vi "AppendTableToReport_Mutation.vi"(0 "Diagram":refnum<vi>, 5 "ObjRef":refnum<vi>, 6 "Kind":string="SubVI", 7 "Information":string="<Not A Path>") -> (3 "Replace?":bool)   [LabVIEW 2020]
uses:
  <vilib>/Utility/Data Type/NI_Data Type.lvlib
  <vilib>/Utility/Data Type/Type Definitions/Data Type.ctl
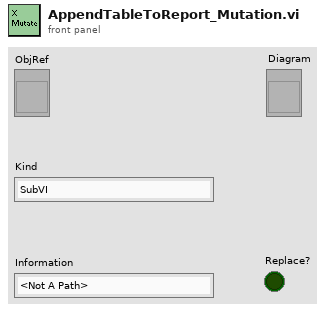
[diagram p1: front panel]
types:
  T1 = typedef "NI_Data Type.lvlib/Data Type.ctl" = enum8{"Invalid Type", "Void", "I8", "I16", "I32", "I64", "U8", "U16", "U32", "U64", "Single Float", "Double Float", "Extended Float", "Single Complex", "Double Complex", "Extended Complex", "Enum U8", "Enum U16", "Enum U32", "Enum U64", "Single Float With Unit", "Double Float With Unit", "Extended Float With Unit", "Single Complex with Unit", "Double Complex with Unit", "Extended Complex with Unit", "Boolean", "String", "Path", "Picture", "Tag", "Array", "Cluster", "Variant", "LV Variant", "Waveform", "Timestamp", "Digital Waveform", "Digital Data", "ExpressData", "Refnum", "External Data", "VI", "Poly VI", "LabVIEW Class Instance", "Fixed Point", "Set Collection", "Map Collection"}
  T2 = typedef "LVPositionTypeDef.ctl" = cluster{"Left":i32, "Top":i32}
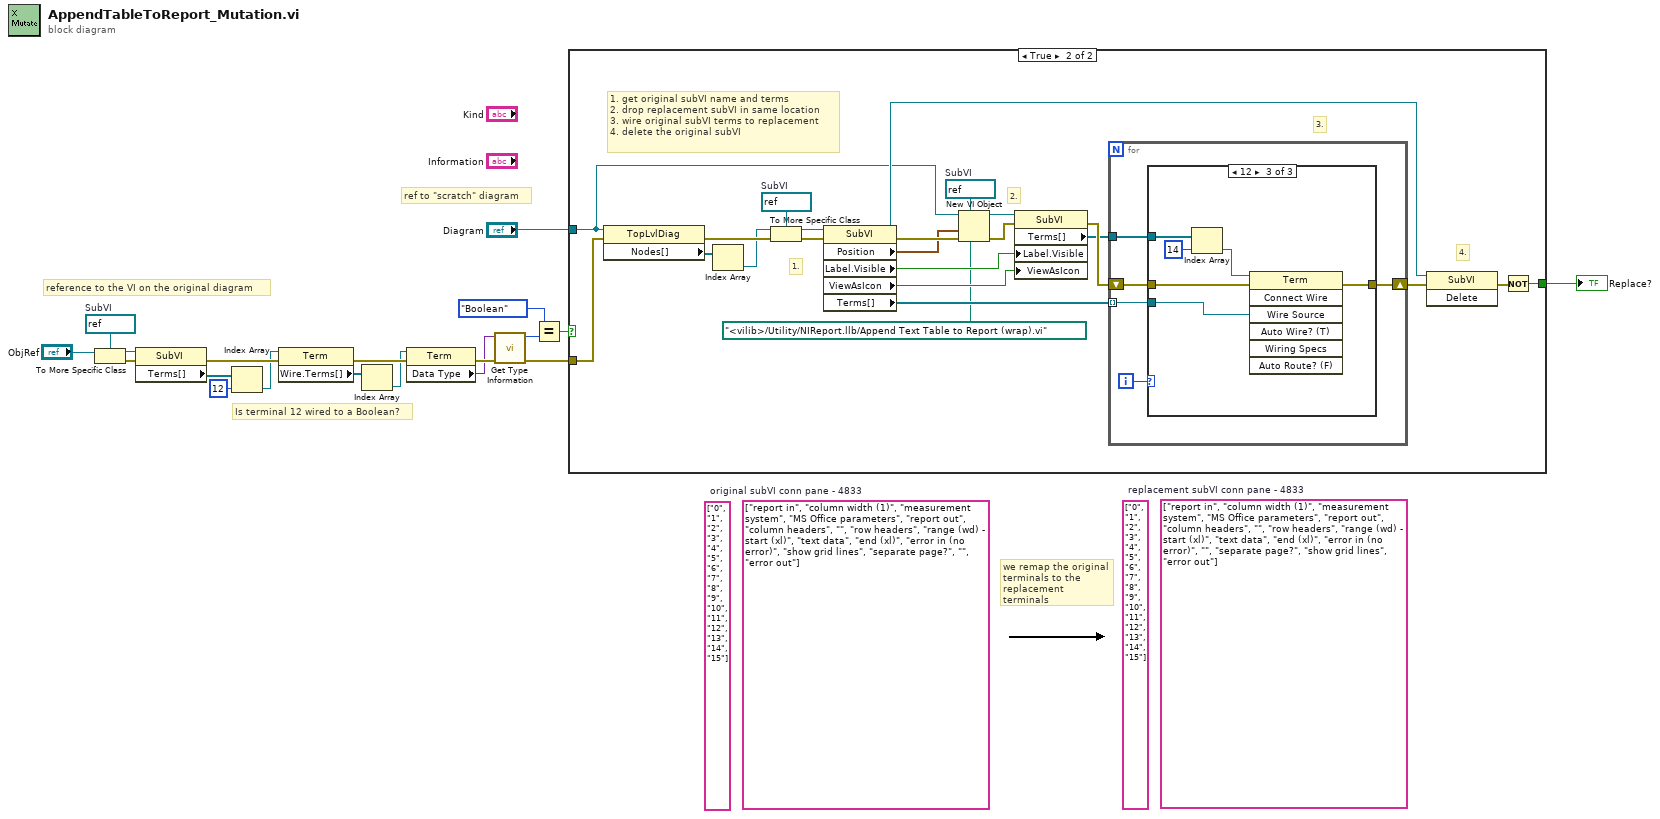
[diagram p0: block diagram]
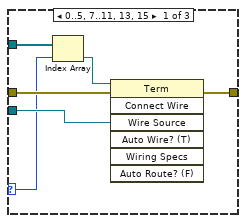
[diagram p3: hidden frame]
diagram:
  w12 = refnum<vi> refnum  # SubVI
  (unwired) string[] ["0", "1", "2", "3", "4", "5", "6", "7", "8", "9", "10", "11", "12", "13", "14", "15"]
  (unwired) string[] ["report in", "column width (1)", "measurement system", "MS Office parameters", "report out", "column headers", "", "row headers", "range (wd) - start (xl)", "text data", "end (xl)", "error in (no error)", "show grid lines", "separate page?", "", "error out"]  # original subVI conn pane - 4833
  (unwired) string[] ["0", "1", "2", "3", "4", "5", "6", "7", "8", "9", "10", "11", "12", "13", "14", "15"]
  (unwired) string[] ["report in", "column width (1)", "measurement system", "MS Office parameters", "report out", "column headers", "", "row headers", "range (wd) - start (xl)", "text data", "end (xl)", "error in (no error)", "", "separate page?", "show grid lines", "error out"]  # replacement subVI conn pane - 4833
  # "Is terminal 12 wired to a Boolean?"
  # "reference to the VI on the original diagram"
  # "we remap the original terminals to the replacement terminals"
  # "ref to \"scratch\" diagram"
  n1 = To More Specific Class(target class=w12, reference="ObjRef") -> (specific class reference=w10:refnum<vi>, error out=w19:errorcluster)  [unwired: 1 in]
  n2 = property class="SubVI"(reference=w10, error in=w19) -> (error out=w18:errorcluster, "Terms[]"=w9:refnum<vi>[])  [unwired: 1 out]
  n3 = Index Array(array=w9, index=12) -> (element=w7:refnum<vi>)
  n4 = property class="Term"(reference=w7, error in=w18) -> (error out=w17:errorcluster, "Wire.Terms[]"=w6:refnum<vi>[])  [unwired: 1 out]
  n5 = Index Array(array=w6) -> (element=w5:refnum<vi>)  [unwired: 1 in]
  n6 = property class="Term"(reference=w5, error in=w17) -> (error out=w16:errorcluster, "Data Type"=w4:variant)  [unwired: 1 out]
  n7 = call <vilib>:"Get Type Information.vi"("error in (no error)"=w16, "variant"=w4) -> ("error out"=w15:errorcluster, "type"=w3:T1)  [unwired: 5 in, 3 out]
  n8 = Equal?(x=Data_Type."Boolean", y=w3) -> (x = y?=w2:bool)
  n9 = case shown="True" w2 {
    tunnel: "Diagram" -> [_ w25]
    tunnel: [_ w24] -> w13
    tunnel: w15 -> [_ w35]
    frame False {
      # "If terminal 7 is not wired to a Boolean we do not need to rewire, because all the other terminals map the same."
    }
    frame True {
      w23 = refnum<vi> refnum  # SubVI
      w34 = refnum<vi> refnum  # SubVI
      # "4."
      # "3."
      # "2."
      # "1."
      # "1. get original subVI name and terms\n2. drop replacement subVI in same location\n3. wire original subVI terms to replacement\n4. delete the original subVI"
      n10 = property class="TopLvlDiag"(reference=w25, error in=w35) -> (error out=w42:errorcluster, "Nodes[]"=w33:refnum<vi>[])  [unwired: 1 out]
      n11 = Index Array(array=w33) -> (element=w32:refnum<vi>)  [unwired: 1 in]
      n12 = To More Specific Class(target class=w34, reference=w32, error in=w42) -> (specific class reference=w26:refnum<vi>, error out=w40:errorcluster)
      n13 = property class="SubVI"(reference=w26, error in=w40) -> (reference out=w30:refnum<vi>, error out=w41:errorcluster, "Position"=w29:T2, "Label.Visible"=w27:bool, "ViewAsIcon"=w28:bool, "Terms[]"=w31:refnum<vi>[])
      n14 = New VI Object(vi object class=w23, owner refnum=w25, position/next to=w29, 6:path "<vilib>/Utility/NIReport.llb/Append Text Table to Report (wrap).vi", 8:w41) -> (object refnum=w20:refnum<vi>, 0:w38:errorcluster)  [unwired: 3 in]
      n15 = property class="SubVI"(reference=w20, error in=w38, "Label.Visible"=w27, "ViewAsIcon"=w28) -> (error out=w37:errorcluster, "Terms[]"=w21:refnum<vi>[])  [unwired: 1 out]
      n16 = for {
        tunnel: w31 -> [w44] mode=indexing
        tunnel: w21 -> [w43]
        shift-right: [w46] -> w39
        shift-left: w37 -> [w47]
        i -> [w45]
        n17 = case shown="12" w45 {
          selector: w45 -> [w48 _ _]
          tunnel: w44 -> [w51 _ w58]
          tunnel: w43 -> [w50 _ w57]
          tunnel: w47 -> [w53 w54 w60]
          tunnel: [w52 w54 w59] -> w46
          frame 0..5, 7..11, 13, 15 {
            n18 = Index Array(array=w50, index=w48) -> (element=w49:refnum<vi>)
            n19 = invoke class="Term" method="Connect Wire"(reference=w49, error in=w53, "Wire Source"=w51) -> (error out=w52:errorcluster)  [unwired: 4 in, 6 out]
          }
          frame 6, 14, Default {
          }
          frame 12 {
            n20 = Index Array(array=w57, index=14) -> (element=w55:refnum<vi>)
            n21 = invoke class="Term" method="Connect Wire"(reference=w55, error in=w60, "Wire Source"=w58) -> (error out=w59:errorcluster)  [unwired: 4 in, 6 out]
          }
        }
      }
      n22 = invoke class="SubVI" method="Delete"(reference=w30, error in=w39) -> (error out=w36:errorcluster)  [unwired: 1 in, 2 out]
      n23 = Not(x=w36) -> (.not. x?=w24:bool)
    }
  }
  "Replace?" <- w13
